vi "Lockin.Low Pass Filter (subVI).vi"(8 "error in (no error)":errorcluster, 9 "Element Data":i32, 10 "signal in":waveform(dbl)[](array[waveform]), 11 "Lockin.DAQ in":refnum<class "Instrument.DAQ.lvclass">) -> (0 "error out":errorcluster, 1 "Fc (Hz)":dbl, 2 "signal out":waveform(dbl)[](array[waveform]))   [LabVIEW 2019, in "Instrument.Lockin.lvlib" / "Instrument.DAQ.lvclass"]
uses:
  Instrument.DAQ.lvclass
  Instrument.DAQ.lvclass/Instrument.DAQ.ctl
  <vilib>/addons/Digital Filter Design/Process.llb/DFD Filtering (Wfm NChan).vi
  <vilib>/addons/Digital Filter Design/NI_DigFilterLicensed.lvlib
panel:
  out "Lockin.DAQ out":refnum<class "Instrument.DAQ.lvclass">
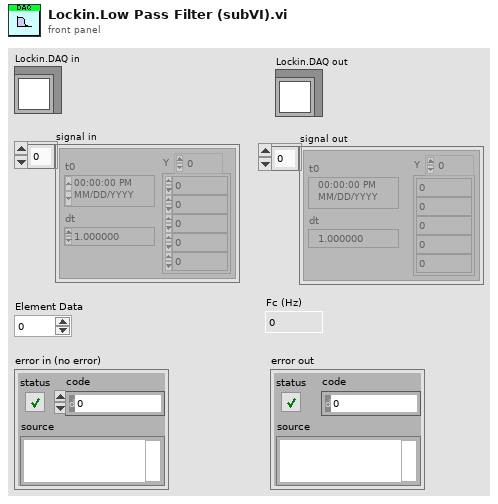
[diagram p1: front panel]
types:
  T1 = typedef "Instrument.Lockin.lvlib/Instrument.DAQ.lvclass/REF.Channel--Cluster--Array.ctl" = T2[]
  T2 = typedef "Instrument.Lockin.lvlib/Instrument.DAQ.lvclass/REF.Channel--Cluster.ctl" = cluster{"Enable?":bool, "Channel":i32, "Frequency":dbl, "Phase":dbl, "TC":dbl, "Roll-Off":i32}
  T3 = typedef "NI_DigFilterLicensed.lvlib/DFD Filter Obj.ctl" = cluster{"mSRate_Fs":dbl, "mSRate_Version":string, "mSRate_Comments":string, "mSRate_OrgCoef":T4, "mSRate_CurCoef":T4, "mSRate_Quantized?":bool, "mSRate_QCoef":T4, "mSRate_QSettings":T6[], "mSRate_Order":i32, "mSRate_Scaling":cluster{"mSRate_ScaleByPowerOf2?":bool, "mSRate_ScaleType":T8}}
  T4 = typedef "NI_DigFilterLicensed.lvlib/DFD Filter Coef.ctl" = cluster{"type":T5, "gain":dbl, "coef a (k)":dbl[], "coef b (v)":dbl[]}
  T5 = typedef "NI_DigFilterLicensed.lvlib/DFD Filter Structure Type Selector.ctl" = enum16{"Undefined", "FIR Direct Form", "FIR Direct Form Transposed", "FIR Symmetric", "FIR Antisymmetric", "IIR Direct Form I", "IIR Direct Form I Transposed", "IIR Direct Form II", "IIR Direct Form II Transposed", "IIR Cascaded Second Order Sections Form I", "IIR Cascaded Second Order Sections Form I Transposed", "IIR Cascaded Second Order Sections Form II", "IIR Cascaded Second Order Sections Form II Transposed", "Lattice Allpass (basic sections)", "Lattice Allpass (one multiplier sections)", "Lattice Allpass (normalized sections)", "Lattice AR (basic sections)", "Lattice AR (one multiplier sections)", "Lattice AR (normalized sections)", "Lattice MA (minimum phase)", "Lattice MA (maximum phase)", "Lattice ARMA (basic sections)", "Lattice ARMA (one multiplier sections)", "Lattice ARMA (normalized sections)"}
  T6 = typedef "NI_DigFilterLicensed.lvlib/dfd_Internal Quantization Settings.ctl" = cluster{"source":T7, "wl":i16, "iwl":i16, "overflow mode":enum16{"Saturation", "Wrap"}, "rounding mode":enum16{"Nearest", "Truncation"}, "signed?":bool}
  T7 = typedef "NI_DigFilterLicensed.lvlib/dfd_Internal Quantization Srcs.ctl" = u16
  T8 = typedef "NI_DigFilterLicensed.lvlib/DFD Coef Norm Type.ctl" = enum16{"No Norm", "Time Domain 1-Norm", "Time Domain 2-Norm", "Time Domain Inf-Norm"}
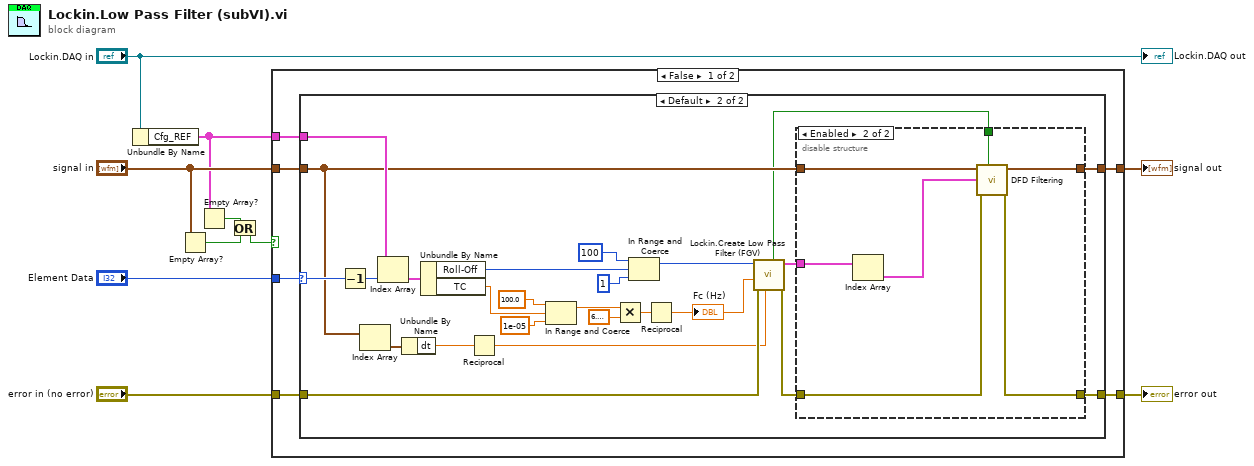
[diagram p0: block diagram]
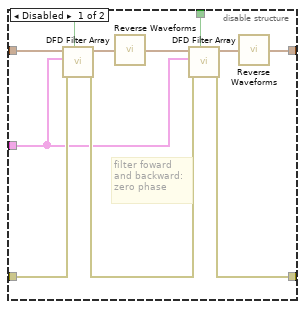
[diagram p3: hidden frame]
diagram:
  n1 = Unbundle By Name("Lockin.DAQ in") -> ("Cfg_REF"=w4:T1)
  n2 = Empty Array?(array="signal in") -> (empty?=w2:bool)
  n3 = Empty Array?(array=w4) -> (empty?=w3:bool)
  n4 = Or(x=w3, y=w2) -> (x .or. y?=w1:bool)
  n5 = case shown="False" w1 {
    tunnel: "error in (no error)" -> [w16 w62]
    tunnel: [w15 w62] -> w9
    tunnel: [w14 w61] -> w8
    tunnel: "Element Data" -> [w12 _]
    tunnel: "signal in" -> [w13 w61]
    tunnel: w4 -> [w11 _]
    frame False {
      n6 = case shown="Default" w12 {
        selector: w12 -> [_ w33]
        tunnel: w16 -> [w18 w27]
        tunnel: [w18 w28] -> w15
        tunnel: w13 -> [w17 w30]
        tunnel: [w17 w29] -> w14
        tunnel: w11 -> [_ w31]
        frame 0 {
        }
        frame Default {
          n7 = Decrement(x=w33) -> (x-1=w32:i32)
          n8 = Index Array(array=w30) -> (element=w43:waveform(dbl))  [unwired: 1 in]
          n9 = Index Array(array=w31, index=w32) -> (element=w42:T2)
          n10 = Unbundle By Name(w43) -> ("dt"=w23:dbl)
          n11 = Unbundle By Name(w42) -> ("Roll-Off"=w20:i32, "TC"=w41:dbl)
          n12 = Reciprocal(x=w23) -> (1/x=w19:dbl)
          n13 = In Range and Coerce(upper limit=100.0, x=w41, lower limit=1e-05) -> (coerced(x)=w34:dbl)  [unwired: 1 out]
          n14 = Multiply(x=w34, y=6.283185307179586) -> (x*y=w38:dbl)
          n15 = In Range and Coerce(upper limit=100, x=w20, lower limit=1) -> (coerced(x)=w26:i32)  [unwired: 1 out]
          n16 = Reciprocal(x=w38) -> (1/x=w24:dbl)
          "Fc (Hz)" <- w24
          n17 = call "Lockin.Create Low Pass Filter (FGV).vi"("fs (Hz)"=w19, "error in (no error)"=w27, "Low Pass Cutoff (Hz)"=w24, "order"=w26) -> ("error out"=w25:errorcluster, "Filters out"=w21:T3[], "init out"=w22:bool)  [unwired: 5 in]
          n18 = disable-structure shown="Enabled" {
            disable-tunnel: w30 -> [w53 w60]
            disable-tunnel: [w49 w58] -> w29
            disable-tunnel: [w48 w56] -> w28
            disable-tunnel: w25 -> [w46 w57]
            disable-tunnel: w22 -> [w45 w59]
            disable-tunnel: w21 -> [w44 w55]
            frame Disabled {
              # "filter foward\nand backward:\nzero phase"
              n19 = call "DFD Filter Array.vi"("init (F)"=w45, "error in (no error)"=w46, "filters"=w44, "signal in"=w53) -> ("error out"=w47:errorcluster, "signal out"=w50:waveform(dbl)[])  [unwired: 6 in]
              n20 = call "Reverse Waveforms.vi"("signal in"=w50) -> ("Array"=w52:waveform(dbl)[])
              n21 = call "DFD Filter Array.vi"("init (F)"=w45, "error in (no error)"=w47, "filters"=w44, "signal in"=w52) -> ("error out"=w48:errorcluster, "signal out"=w51:waveform(dbl)[])  [unwired: 6 in]
              n22 = call "Reverse Waveforms.vi"("signal in"=w51) -> ("Array"=w49:waveform(dbl)[])
            }
            frame Enabled {
              n23 = Index Array(array=w55) -> (element=w54:T3)  [unwired: 1 in]
              n24 = call-poly <vilib>:"DFD Filtering.vi"("init? (F)"=w59, "error in (no error)"=w57, "filter"=w54, "signal in"=w60) -> ("error out"=w56:errorcluster, "signal out"=w58:waveform(dbl)[])  [unwired: 6 in]
            }
          }
        }
      }
    }
    frame True {
    }
  }
  "error out" <- w9
  "signal out" <- w8
  "Lockin.DAQ out" <- "Lockin.DAQ in"
